vi "CompareLastHWI_Novatech.vi"(9 "Last Novatech HWI":T1 {"Hardware Image"."3 phase" format="%#.5f"; "Hardware Image"."2 phase" format="%#.5f"; "Hardware Image"."3 Power [dBm]" format="%#.5f"; "Hardware Image"."3 Freq. [MHz]" format="%#_5e"; "Hardware Image"."2 Power [dBm]" format="%#.5f"; "Hardware Image"."2 Freq. [MHz]" format="%#_5e"}, 10 "Novatech HWI":T1 {"Hardware Image"."3 phase" format="%#.5f"; "Hardware Image"."2 phase" format="%#.5f"; "Hardware Image"."3 Power [dBm]" format="%#.5f"; "Hardware Image"."3 Freq. [MHz]" format="%#_5e"; "Hardware Image"."2 Power [dBm]" format="%#.5f"; "Hardware Image"."2 Freq. [MHz]" format="%#_5e"}) -> (1 "Skip":i32[](array[numeric]), 2 "change?":bool)   [LabVIEW 2013]
doc: "Compare all Novatech hardware info (COM port and HWI) and return \"change?\" boolean if anything changes. Additionally, since Novatechs can be programmed line-by-line, output \"Skip\" array which denotes which Tabled lines (ch 0/1) need to be programmed."
uses:
  Utils/Unequal_safe/Unequal_Safe_2dU16.vi
  Utils/Unequal_safe/Unequal_Safe_2dDBL.vi
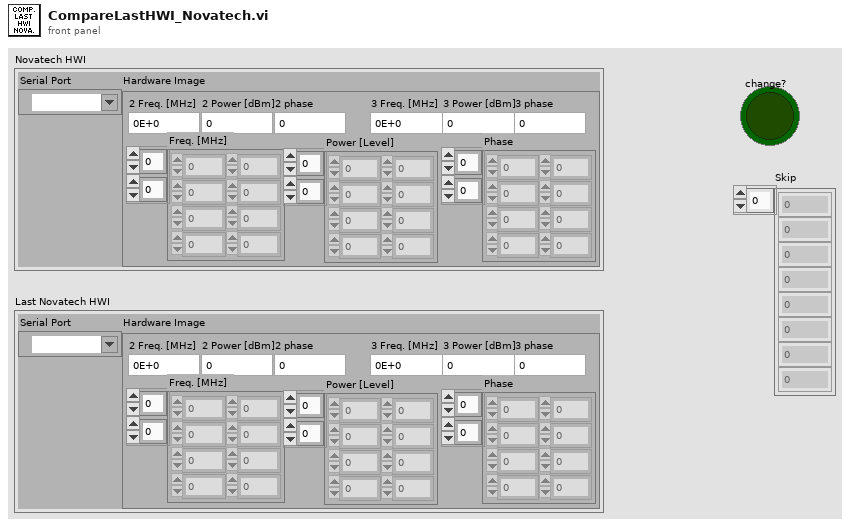
[diagram p1: front panel]
types:
  T1 = cluster{"Serial Port":refnum<visa-resource-name>, "Hardware Image":cluster{"Freq. [MHz]":dbl[][], "Power [Level]":u16[][], "Phase":u16[][], "2 Freq. [MHz]":dbl, "2 Power [dBm]":u16, "2 phase":u16, "3 Freq. [MHz]":dbl, "3 Power [dBm]":u16, "3 phase":u16}}
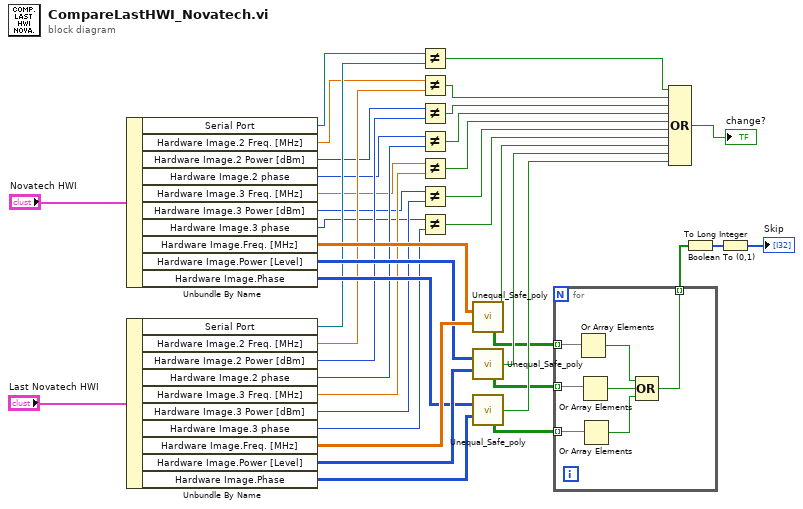
[diagram p0: block diagram]
diagram:
  n1 = Unbundle By Name("Novatech HWI") -> ("Serial Port"=w21:refnum<visa-resource-name>, "Hardware Image.2 Freq. [MHz]"=w13:dbl, "Hardware Image.2 Power [dBm]"=w12:u16, "Hardware Image.2 phase"=w11:u16, "Hardware Image.3 Freq. [MHz]"=w10:dbl, "Hardware Image.3 Power [dBm]"=w9:u16, "Hardware Image.3 phase"=w8:u16, "Hardware Image.Freq. [MHz]"=w28:dbl[][], "Hardware Image.Power [Level]"=w29:u16[][], "Hardware Image.Phase"=w30:u16[][])
  n2 = Unbundle By Name("Last Novatech HWI") -> ("Serial Port"=w20:refnum<visa-resource-name>, "Hardware Image.2 Freq. [MHz]"=w14:dbl, "Hardware Image.2 Power [dBm]"=w15:u16, "Hardware Image.2 phase"=w16:u16, "Hardware Image.3 Freq. [MHz]"=w17:dbl, "Hardware Image.3 Power [dBm]"=w18:u16, "Hardware Image.3 phase"=w19:u16, "Hardware Image.Freq. [MHz]"=w33:dbl[][], "Hardware Image.Power [Level]"=w32:u16[][], "Hardware Image.Phase"=w31:u16[][])
  n3 = Not Equal?(x=w21, y=w20) -> (x != y?=w7:bool)
  n4 = Not Equal?(x=w13, y=w14) -> (x != y?=w6:bool)
  n5 = Not Equal?(x=w12, y=w15) -> (x != y?=w5:bool)
  n6 = Not Equal?(x=w11, y=w16) -> (x != y?=w4:bool)
  n7 = Not Equal?(x=w10, y=w17) -> (x != y?=w2:bool)
  n8 = Not Equal?(x=w9, y=w18) -> (x != y?=w1:bool)
  n9 = Not Equal?(x=w8, y=w19) -> (x != y?=w3:bool)
  n10 = call-poly "Unequal_Safe_poly.vi"("x"=w28, "y"=w33) -> ("Diff?"=w38:bool, "Diff? array"=w27:bool[][])  [unwired: 12 in]
  n11 = call-poly "Unequal_Safe_poly.vi"("x"=w29, "y"=w32) -> ("Diff?"=w37:bool, "Diff? array"=w26:bool[][])  [unwired: 12 in]
  n12 = call-poly "Unequal_Safe_poly.vi"("x"=w30, "y"=w31) -> ("Diff?"=w36:bool, "Diff? array"=w25:bool[][])  [unwired: 12 in]
  n13 = for {
    tunnel: w27 -> [w46] mode=indexing
    tunnel: w26 -> [w45] mode=indexing
    tunnel: w25 -> [w44] mode=indexing
    tunnel: [w40] -> w24 mode=indexing
    n14 = Or Array Elements(Boolean array=w46) -> (logical OR=w42:bool)
    n15 = Or Array Elements(Boolean array=w45) -> (logical OR=w43:bool)
    n16 = Or Array Elements(Boolean array=w44) -> (logical OR=w41:bool)
    n17 = Compound Arithmetic op=OR(w42, w43, w41) -> (w40:bool)
  }
  n18 = Compound Arithmetic op=OR(w7, w6, w5, w4, w2, w1, w3, w38, w37, w36) -> (→"change?":bool)
  n19 = Boolean To (0,1)(Boolean=w24) -> (0, 1=w23:i16[])
  n20 = To Long Integer(number=w23) -> (32bit integer=→"Skip":i32[])
